vi "Clear Fault.vi"(8 "error in":errorcluster, 9 "timeout (-1)":i32=-1, 10 "code (0 for all)":i32, 11 "Standard Engine Runtime in":refnum<class "Standard Engine Runtime.lvclass">) -> (0 "error out":errorcluster, 3 "Standard Engine Runtime out":refnum<class "Standard Engine Runtime.lvclass">)   [LabVIEW 2013, in "Standard Engine Runtime.lvclass"]
doc: "Clears the record of a fault in the engine."
uses:
  Standard Engine Runtime.lvclass
  Standard Engine Runtime.lvclass/Standard Engine Runtime.ctl
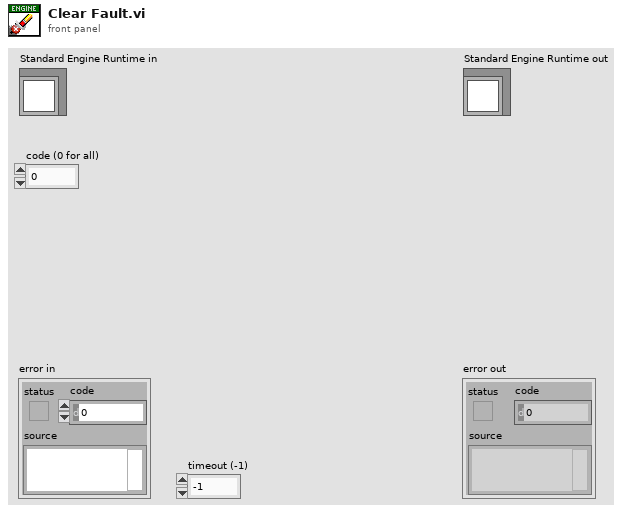
[diagram p1: front panel]
types:
  T1 = typedef "Engine Runtime Interface.lvclass/Fault.ctl" = cluster{"code":i32, "error classification":T2, "Source GUID":string, "first reported time":timestamp, "number reported":u32, "last reported time":timestamp}
  T2 = typedef "TBM module execution interface.lvclass/error classification.ctl" = enum16{"unknown", "none", "trivial", "recoverable", "critical"}
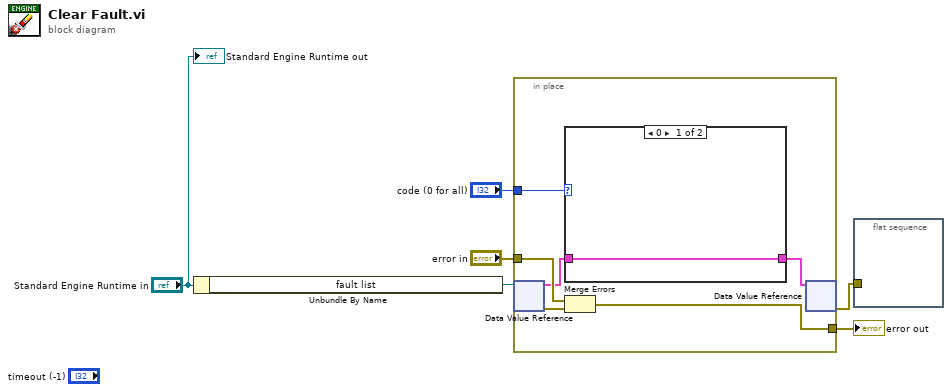
[diagram p0: block diagram]
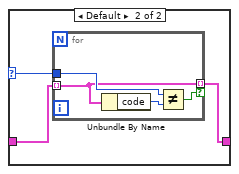
[diagram p2: hidden frame]
diagram:
  n1 = Unbundle By Name("Standard Engine Runtime in") -> ("fault list"=w6:refnum<data-value>)
  n2 = in-place {
    in-place-border: "error in" -> [w12]
    in-place-border: [w10] -> w3
    in-place-border: "code (0 for all)" -> [w7]
    n3 = in-place-dvr #1(w6) -> (w9:T1[], w11:errorcluster)
    n4 = case shown="0" w7 {
      selector: w7 -> [_ w14]
      tunnel: w9 -> [w13 w16]
      tunnel: [w13 w15] -> w8
      frame 0 {
      }
      frame Default {
        n5 = for {
          tunnel: w16 -> [w18] mode=indexing
          tunnel: w14 -> [w19]
          tunnel: [w18] -> w15 mode=indexing if=w17
          n6 = Unbundle By Name(w18) -> ("code"=w20:i32)
          n7 = Not Equal?(x=w19, y=w20) -> (x != y?=w17:bool)
        }
      }
    }
    n8 = Merge Errors(w12, w11) -> (w10:errorcluster)
    n9 = in-place-dvr #1(w8) -> (w5:errorcluster)  [unwired: 1 out]
  }
  "error out" <- w3
  n10 = flat-sequence {
    tunnel: w5 -> [_]
    frame #0 {
    }
  }
  "Standard Engine Runtime out" <- "Standard Engine Runtime in"
